vi "Read Property names.vi"(8 "error in (no error)":errorcluster, 11 "Metadata in":refnum<class "Metadata.lvclass">) -> (0 "error out":errorcluster, 2 "Property names":string[](array[string]), 3 "Metadata out":refnum<class "Metadata.lvclass">)   [LabVIEW 2020, in "Metadata.lvclass"]
uses:
  Metadata.lvclass
  Metadata.lvclass/Metadata.ctl
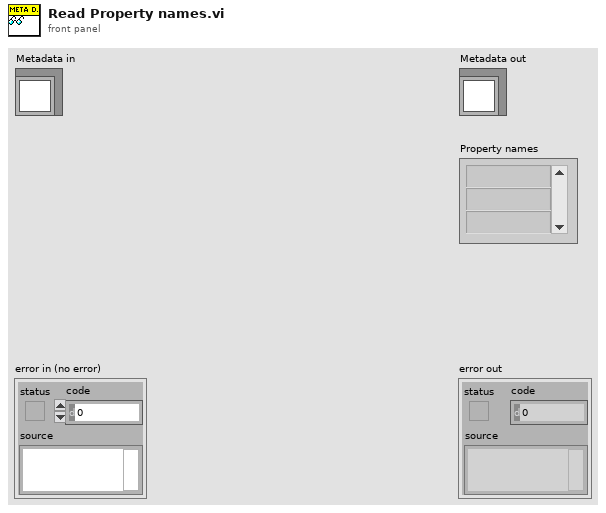
[diagram p1: front panel]
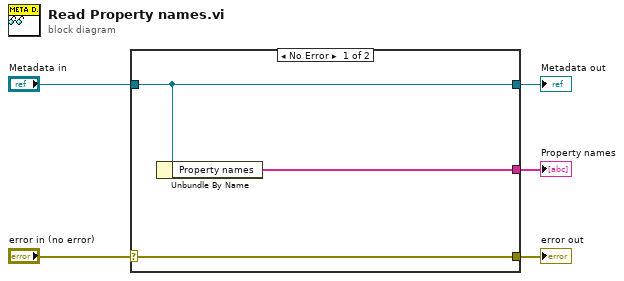
[diagram p0: block diagram]
diagram:
  n1 = case shown="No Error" "error in (no error)" {
    selector: "error in (no error)" -> [w8 w9]
    tunnel: [w8 w9] -> w4
    tunnel: [w7 w10] -> w2
    tunnel: "Metadata in" -> [w7 w10]
    tunnel: [w6 _] -> w1
    frame No Error {
      n2 = Unbundle By Name(w7) -> ("Property names"=w6:string[])
    }
    frame Error {
    }
  }
  "error out" <- w4
  "Metadata out" <- w2
  "Property names" <- w1
